vi "Get Connections - 1Pin MConn.vi"(6 "pin type":T1, 8 "error in":errorcluster, 9 "site":i32=-1, 10 "pin or relay name":string, 11 "session reservation in":refnum<class "Session Reservation.lvclass">) -> (0 "error out":errorcluster, 2 "connections":T2[](array[typedef]), 3 "session reservation out":refnum<class "Session Reservation.lvclass">)   [LabVIEW 2020, in "Plug-In SDK niDMM Sessions.lvlib"]
doc: "Gets the NI-DMM connection information for the given <b>pin type</b>, <b>pin or relay name</b>, and <b>site</b>. If the <b>pin or relay name</b> input is unwired, the connection information for all pins on the given <b>site</b> will be returned. If the <b>site</b> input is unwired, the connection information for the given <b>pin or relay name</b> for all sites will be returned. If both the <b>pin or relay name</b> and <b>site</b> inputs are unwired, the connection information for all pins and on all sites will be returned.\n\nIf you have not called <b>Create Sessions.vi</b> prior to calling this VI, the connection information will be returned with the correct information but will have an invalid session."
uses:
  Plug-In SDK niDMM Sessions.lvlib
  f7b4a7e6-b913-4a56-832a-4a2a9d963d9c.vi
  Clients/Session Management V1/Session Reservation/Connection.ctl
  Clients/Session Management V1/Session Reservation/Session Reservation.lvclass
  Connection with Session.ctl
  Session Factory/Session Factory.lvclass
  Clients/Session Management V1/Session Reservation/Pin Type.ctl
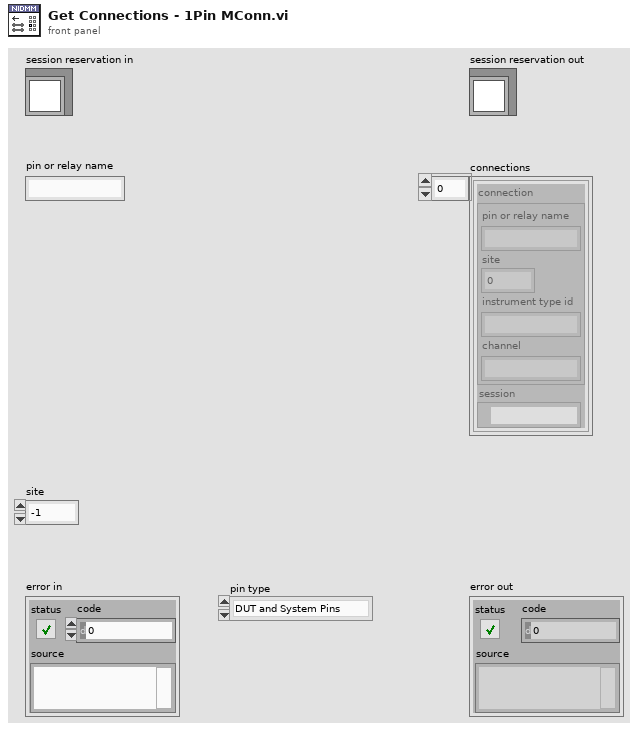
[diagram p1: front panel]
types:
  T1 = typedef "NI Session Management V1 Client.lvlib/Session Reservation.lvclass/Pin Type.ctl" = enum16{"DUT and System Pins", "System Pins"}
  T2 = typedef "Plug-In SDK niDMM Sessions.lvlib/Connection with Session.ctl" = cluster{"connection":T3, "session":refnum<k15>}
  T3 = typedef "NI Session Management V1 Client.lvlib/Session Reservation.lvclass/Connection.ctl" = cluster{"pin or relay name":string, "site":i32, "instrument type id":string, "channel":string}
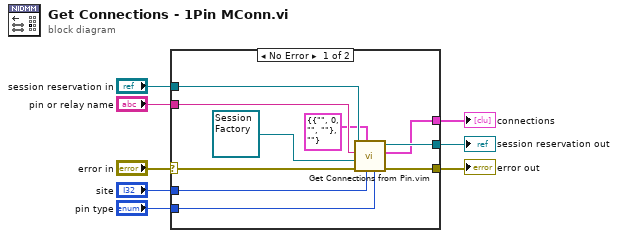
[diagram p0: block diagram]
diagram:
  n1 = case shown="No Error" "error in" {
    selector: "error in" -> [w12 w19]
    tunnel: "session reservation in" -> [w15 w20]
    tunnel: "pin or relay name" -> [w13 _]
    tunnel: [w16 w19] -> w5
    tunnel: [w18 w20] -> w4
    tunnel: [w17 _] -> w2
    tunnel: "site" -> [w14 _]
    tunnel: "pin type" -> [w9 _]
    frame No Error {
      n2 = call "Get Connections from Pin.vim"("pin type"=w9, "site"=w14, "connection type"=T2 {"connection"={"pin or relay name"="", "site"=0, "instrument type id"="", "channel"=""}, "session"=""} ("niDMM connection"), "error in"=w12, "session factory"=refnum<class "Session Factory.lvclass"> refnum ("MeasurementLink niDMM.lvlib:Instrument.lvclass"), "pin or relay name"=w13, "session reservation in"=w15) -> ("error out"=w16:errorcluster, "connections"=w17:T2[], "session reservation out"=w18:refnum<class "Session Reservation.lvclass">)  [unwired: 2 in]
    }
    frame Error {
    }
  }
  "error out" <- w5
  "session reservation out" <- w4
  "connections" <- w2
